vi "json allocate token.vi"(7 "type":T1, 8 "token count in":i32, 9 "start":i32, 10 "parent token":i32, 11 "tokens in":T2[](array[typedef])) -> (0 "token count out":i32, 2 "current token out":i32, 3 "tokens out":T2[](array[typedef]))   [LabVIEW 2013]
uses:
  json token.ctl
  json node type.ctl
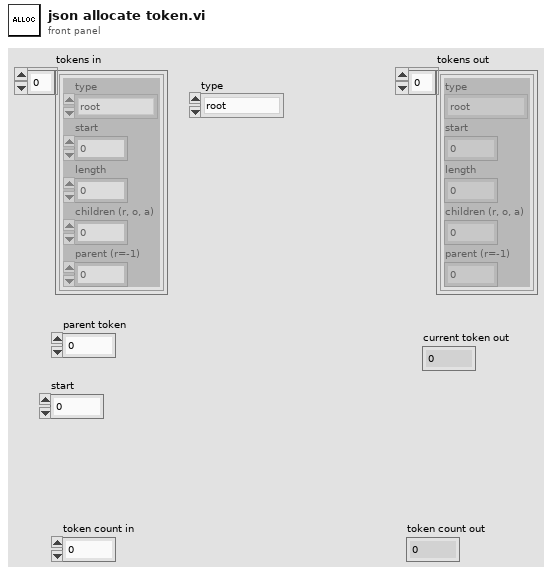
[diagram p1: front panel]
types:
  T1 = typedef "json node type.ctl" = enum16{"root", "object", "array", "number", "string value", "string key", "true", "false", "null"}
  T2 = typedef "json token.ctl" = cluster{"type":T1, "start":i32, "length":i32, "children (r, o, a)":u16, "parent (r=-1)":i32}
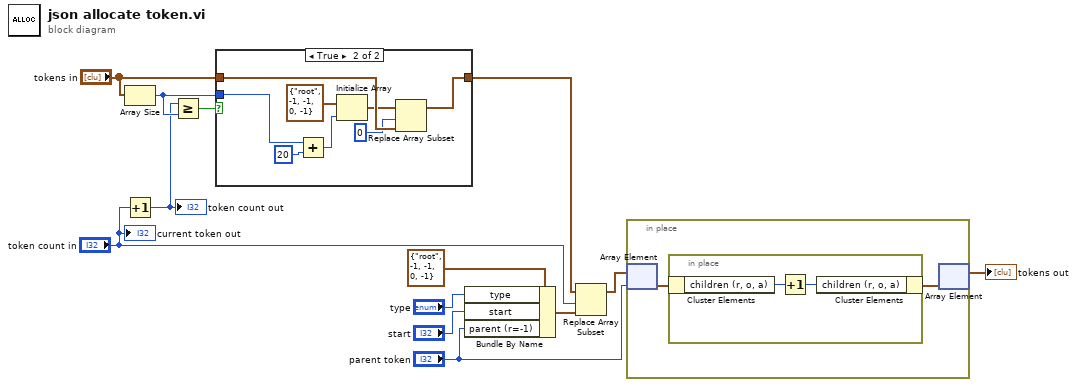
[diagram p0: block diagram]
diagram:
  n1 = Array Size(array="tokens in") -> (size(s)=w9:i32)
  n2 = Increment(x="token count in") -> (x+1=w8:i32)
  "token count out" <- w8
  n3 = Greater Or Equal?(x=w8, y=w9) -> (x >= y?=w13:bool)
  n4 = case shown="True" w13 {
    tunnel: "tokens in" -> [w14 w20]
    tunnel: [w14 w21] -> w12
    tunnel: w9 -> [_ w22]
    frame False {
    }
    frame True {
      n5 = Add(x=w22, y=20 ("dimension size")) -> (x+y=w18:i32)
      n6 = Initialize Array(T2 {"type"=enum."root", "start"=-1, "length"=-1, "children (r, o, a)"=0, "parent (r=-1)"=-1} ("token 2"), w18) -> (w16:T2[])
      n7 = Replace Array Subset(array=w16, new element=w20, index=0) -> (w21:T2[])
    }
  }
  n8 = Bundle By Name(cluster=T2 {"type"=enum."root", "start"=-1, "length"=-1, "children (r, o, a)"=0, "parent (r=-1)"=-1} ("token 2"), "type"="type", "start"="start", "parent (r=-1)"="parent token") -> (w6:T2)
  n9 = Replace Array Subset(array=w12, new element=w6, index="token count in") -> (w3:T2[])
  n10 = in-place {
    n11 = in-place-array #1(w3, "parent token") -> (w24:T2)
    n12 = in-place {
      n13 = in-place-cluster #2(w24) -> ("children (r, o, a)"=w26:u16)
      n14 = Increment(x=w26) -> (x+1=w25:u16)
      n15 = in-place-cluster #2("children (r, o, a)"=w25) -> (w23:T2)
    }
    n16 = in-place-array #1(w23) -> (→"tokens out":T2[])  [unwired: 1 out]
  }
  "current token out" <- "token count in"
